vi "initImageAll.vi"() -> (3 "Refnum out":T1)   [LabVIEW 2011, in "MagAnalysis_Online.lvclass"]
uses:
  MagAnalysis_Online.lvclass
  IMAQ Image.ctl
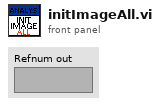
[diagram p1: front panel]
types:
  T1 = typedef "IMAQ Image.ctl" = refnum<image>
  T2 = typedef "Image Type" = u32
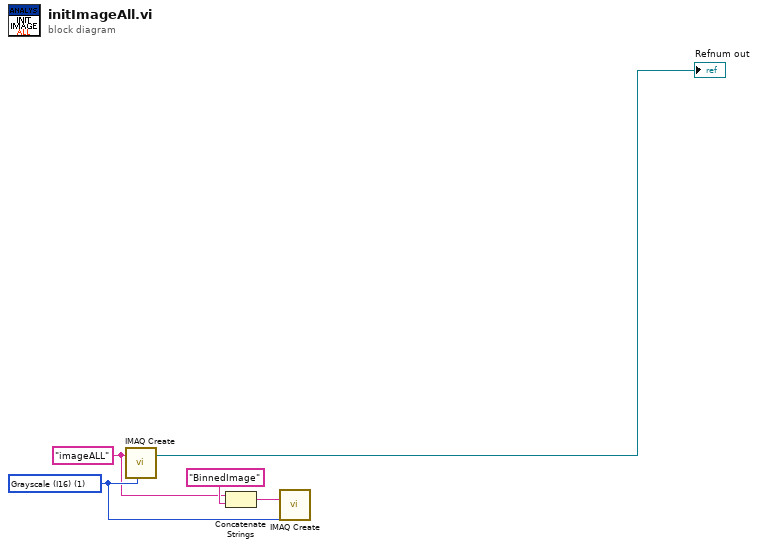
[diagram p0: block diagram]
diagram:
  w5 = T2 1 items=["Grayscale (U8)", "Grayscale (I16)", "Grayscale (SGL)", "Complex (CSG)", "RGB (U32)", "HSL (U32)", "RGB (U64)", "Grayscale (U16)"] ("Image Type")
  w2 = "imageALL" ("Image Name")
  n1 = call "IMAQ Create"("Image Name"=w2, "Image Type"=w5) -> ("New Image"=→"Refnum out":T1)  [unwired: 3 in, 1 out]
  n2 = Concatenate Strings(w2, "BinnedImage") -> (w4:string)
  n3 = call "IMAQ Create"("Image Name"=w4, "Image Type"=w5) -> ()  [unwired: 3 in, 2 out]
